vi "EventServer_Monitor App.vi"() -> ()   [LabVIEW 2018]
panel:
  in  "Unhandled Events":i32(listbox)
  in  "Subscribed Events":i32(listbox)
  in  "Registered Clients":i32(listbox)
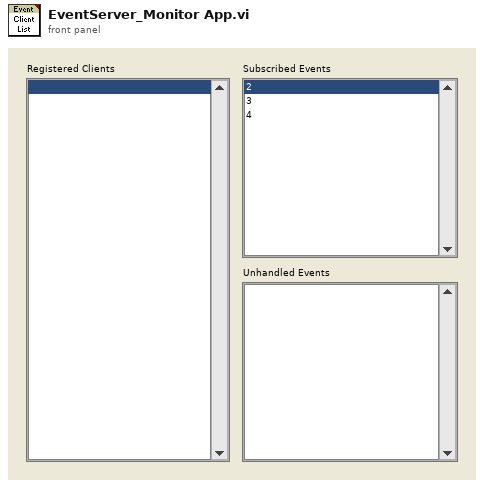
[diagram p1: front panel]
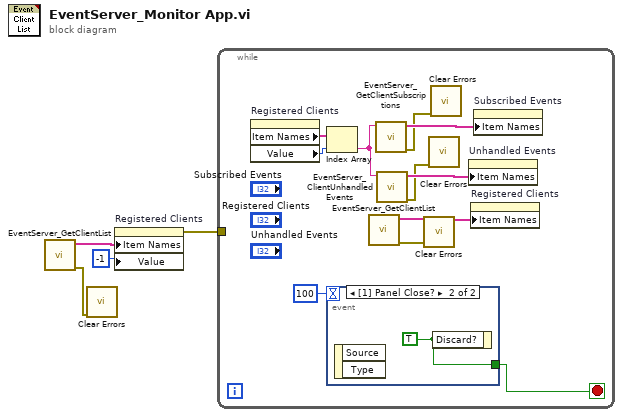
[diagram p0: block diagram]
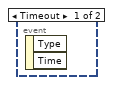
[diagram p2: hidden frame]
diagram:
  n1 = call "EventServer_GetClientList.vi"() -> ("error out"=w1:errorcluster, "Client List"=w2:string[])  [unwired: 1 in, 9 out]
  n2 = call <vilib>:"Clear Errors.vi"("error in (no error)"=w1) -> ()  [unwired: 1 in, 6 out]
  n3 = property on="Registered Clients" class="LstBox (strict)"("Item Names"=w2, "Value"=-1 ("Subscribed Events")) -> (error out=w3:errorcluster)  [unwired: 2 in, 1 out]
  n4 = while {
    tunnel: w3 -> [_]
    stop <- w8 stop-if-true
    n5 = property on="Registered Clients" class="LstBox (strict)"() -> ("Item Names"=w15:string[], "Value"=w14:i32)  [unwired: 2 in, 2 out]
    n6 = Index Array(array=w15, index=w14) -> (element=w13:string)
    n7 = event shown="[1] Panel Close?" {
      selector: _ -> [_ _]
      dyn-events: _ -> [_ _]
      timeout: 100 -> [_ _]
      tunnel: [_ w16] -> w8
      event Timeout {
        n8 = event-data() -> ()  [unwired: 3 out]
      }
      event Panel Close? {
        w16 = TRUE ("Discard?")
        n9 = event-data() -> ()  [unwired: 3 out]
        n10 = event-data("Discard?"=w16) -> ()  [unwired: 1 in, 1 out]
      }
    }
    n11 = call "EventServer_GetClientList.vi"() -> ("error out"=w5:errorcluster, "Client List"=w10:string[])  [unwired: 1 in, 9 out]
    n12 = call "EventServer_GetClientSubscriptions.vi"("Client Name"=w13) -> ("error out"=w7:errorcluster, "Subscription"=w12:string[])  [unwired: 1 in, 8 out]
    n13 = call "EventServer_ClientUnhandledEvents.vi"("Client Name"=w13) -> ("error out"=w6:errorcluster, "Subscription"=w11:string[])  [unwired: 1 in, 8 out]
    n14 = call <vilib>:"Clear Errors.vi"("error in (no error)"=w5) -> ()  [unwired: 1 in, 6 out]
    n15 = call <vilib>:"Clear Errors.vi"("error in (no error)"=w6) -> ()  [unwired: 1 in, 6 out]
    n16 = call <vilib>:"Clear Errors.vi"("error in (no error)"=w7) -> ()  [unwired: 1 in, 6 out]
    n17 = property on="Unhandled Events" class="LstBox (strict)"("Item Names"=w11) -> ()  [unwired: 2 in, 2 out]
    n18 = property on="Registered Clients" class="LstBox (strict)"("Item Names"=w10) -> ()  [unwired: 2 in, 2 out]
    n19 = property on="Subscribed Events" class="LstBox (strict)"("Item Names"=w12) -> ()  [unwired: 2 in, 2 out]
  }
